vi "Generate Simulated Data.vi"(6 "Acquisition":refnum<queue>, 8 "error in (no error)":errorcluster, 11 "Data Stream":dbl[](array[numeric])) -> (0 "error out":errorcluster, 2 "Data Out":variant[](array[variant]), 3 "Disconnected":bool=TRUE)   [LabVIEW 2022 SP3, in "Acquisition.lvlib"]
doc: "Generates sample waveforms according to the signal type in the HW Config input."
uses:
  Acquisition.lvlib
  support/Message Queue/Message Cluster.ctl
  <vilib>/Analysis/2dsp.llb/2D Convolution (DBL).vi
  support/Message Queue/Enqueue Message (Single).vi
  GlobalVariable/GlobalPowerByTime.vi
  GlobalVariable/GlobalSet0.vi
  GlobalVariable/GlobalPosYbyTime.vi
  GlobalVariable/GlobalPosXbyTime.vi
  GlobalVariable/GlobalProfileByTime.vi
  GlobalVariable/Globalt0.vi
  GlobalVariable/GlobalTensionByTime.vi
  GlobalVariable/GlobalTemperatureByTime.vi
  GlobalVariable/GlobalTimeStep.vi
  <vilib>/gmath/interp.llb/Create Mesh Grid (2D) (x,y arrays).vi
  support/Message Queue/Message Queue.lvlib
  <vilib>/gmath/NI_Gmath.lvlib
  <vilib>/Analysis/NI_AALPro.lvlib
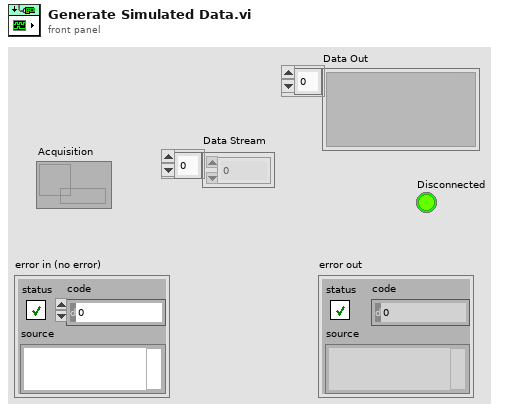
[diagram p1: front panel]
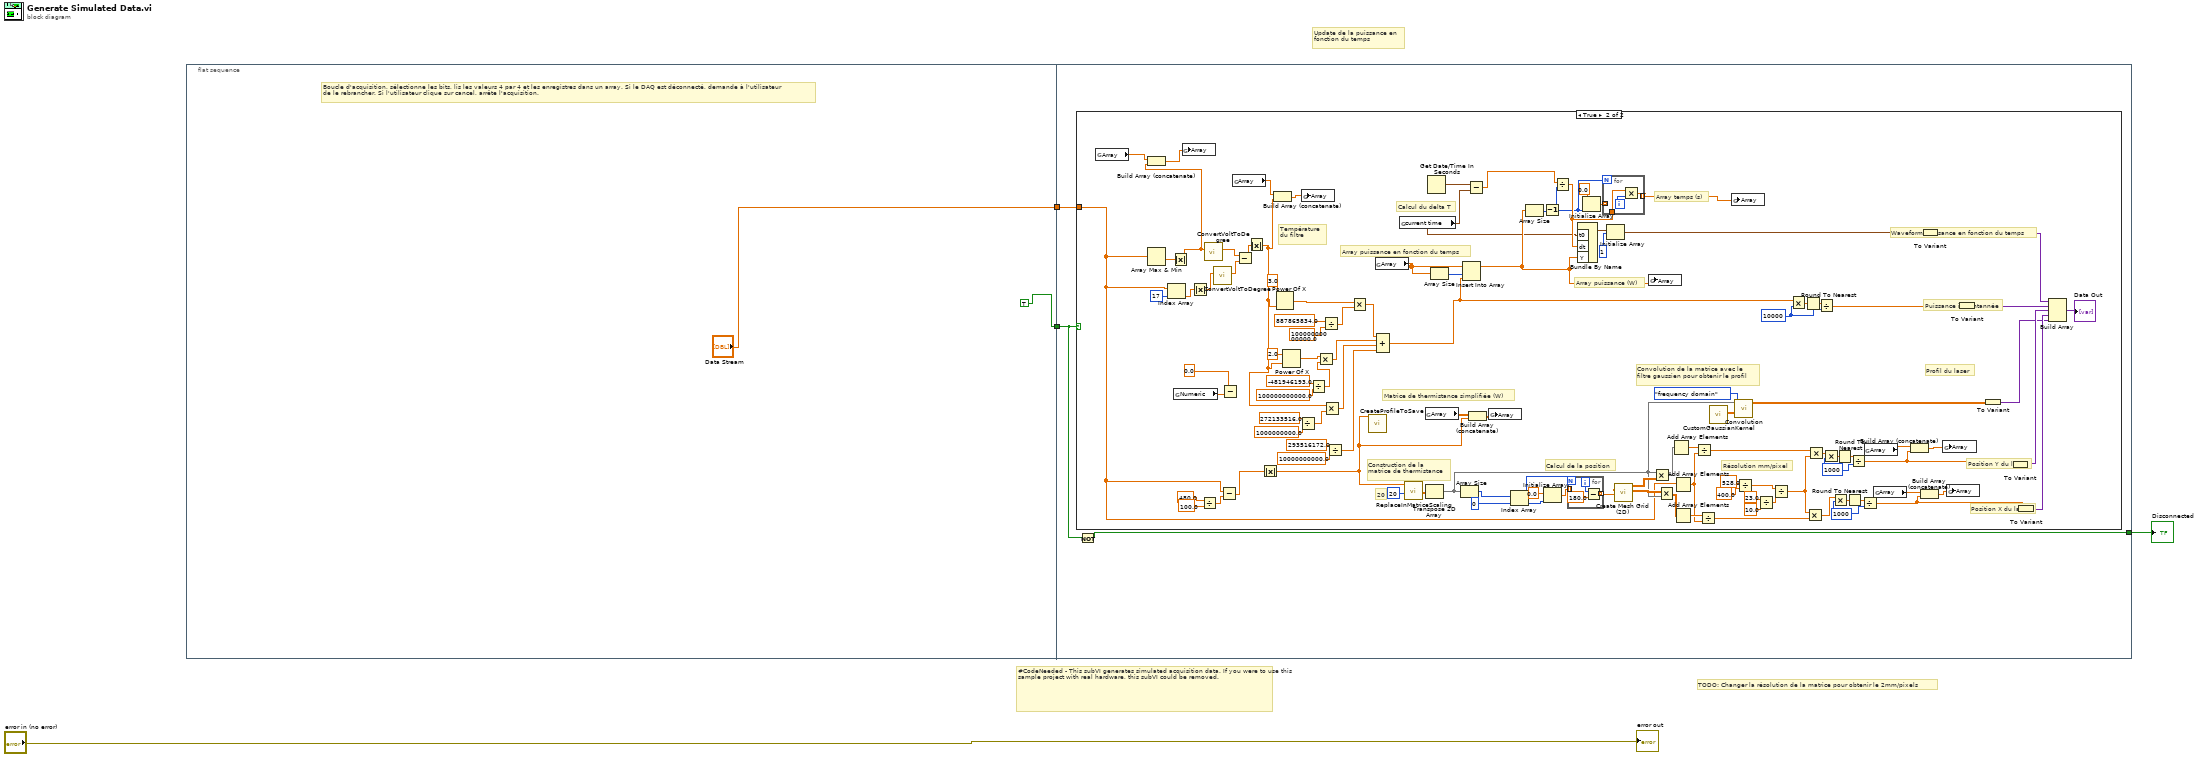
[diagram p0: block diagram]
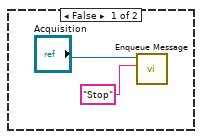
[diagram p2: hidden frame]
diagram:
  # "TODO: Changer la résolution de la matrice pour obtenir le 2mm/pixels"
  # "Update de la puissance en\nfonction du temps"
  # "#CodeNeeded - This subVI generates simulated acquisition data. If you were to use this sample project with real hardware, this subVI could be removed."
  n1 = flat-sequence {
    tunnel: [TRUE] -> w3
    tunnel: ["Data Stream"] -> w1
    tunnel: w3 -> [w7]
    tunnel: [w9] -> w2
    tunnel: w1 -> [w8]
    frame #0 {
      # "Boucle d'acquisition, sélectionne les bits, lis les valeurs 4 par 4 et les enregistres dans un array. Si le DAQ est déconnecté, demande à l'utilisateur \nde le rebrancher. Si l'utilisateur clique sur cancel, arrête l'acquisition."
    }
    frame #1 {
      n2 = case shown="True" w7 {
        tunnel: w8 -> [_ w42]
        frame False {
          n3 = call-poly "Enqueue Message.vi"("Message"="Stop", "Message Queue"="Acquisition") -> ()  [unwired: 8 in, 2 out]
        }
        frame True {
          w79 = 1000
          w83 = 1000
          w89 = 10000
          # "20"
          # "Résolution mm/pixel"
          # "Calcul du delta T"
          # "Matrice de thermistance simplifiée (W)"
          # "Température \ndu filtre"
          # "Calcul de la position"
          # "Construction de la \nmatrice de thermistance"
          # "Position X du laser"
          # "Position Y du laser"
          # "Profil du laser"
          # "Puissance instantannée"
          # "Waveform puissance en fonction du temps"
          # "Array puissance (W)"
          # "Array temps (s)"
          # "Convolution de la matrice avec le \nfiltre gaussien pour obtenir le profil"
          # "Array puissance en fonction du temps"
          n4 = global read "GlobalTensionByTime.vi" "Array"() -> (w59:dbl[])
          n5 = Array Max & Min(array=w42) -> (min value=w18:dbl)  [unwired: 3 out]
          n6 = Index Array(array=w42, index=17) -> (element=w17:dbl)
          n7 = Absolute Value(x=w18) -> (abs(x)=w41:dbl)
          n8 = Build Array (concatenate)(w59, w41) -> (w58:dbl[])
          n9 = global read "GlobalSet0.vi" "Numeric"() -> (w20:dbl)
          n10 = global write "GlobalTensionByTime.vi" "Array"(w58) -> ()
          n11 = Absolute Value(x=w17) -> (abs(x)=w16:dbl)
          n12 = Divide(x=480.0, y=100.0) -> (x/y=w48:dbl)
          n13 = call "ConvertVoltToDegree.vi"("Tension"=w41) -> ("Température"=w14:dbl)  [unwired: 10 in]
          n14 = call "ConvertVoltToDegree.vi"("Tension"=w16) -> ("Température"=w15:dbl)  [unwired: 10 in]
          n15 = Subtract(x=w42, y=w48) -> (x-y=w47:dbl[])
          n16 = Subtract(x=0.0, y=w20) -> ()  [unwired: 1 out]
          n17 = global read "GlobalTemperatureByTime.vi" "Array"() -> (w56:dbl[])
          n18 = Subtract(x=w14, y=w15) -> (x-y=w13:dbl)
          n19 = Absolute Value(x=w13) -> (abs(x)=w12:dbl)
          n20 = Absolute Value(x=w47) -> (abs(x)=w46:dbl[])
          n21 = Build Array (concatenate)(w56, w12) -> (w57:dbl[])
          n22 = Power Of X(1:w12, 2:3.0 ("y")) -> (0:w38:dbl)
          n23 = Power Of X(1:w12, 2:2.0 ("y")) -> (0:w32:dbl)
          n24 = Divide(x=272133516.0, y=1000000000.0) -> (x/y=w27:dbl)
          n25 = global write "GlobalTemperatureByTime.vi" "Array"(w57) -> ()
          n26 = Divide(x=-481946193.0, y=100000000000.0) -> (x/y=w31:dbl)
          n27 = Multiply(x=w32, y=w31) -> (x*y=w29:dbl)
          n28 = Divide(x=887865834.0, y=10000000000000.0) -> (x/y=w37:dbl)
          n29 = Multiply(x=w12, y=w27) -> (x*y=w26:dbl)
          n30 = Divide(x=293516172.0, y=10000000000.0) -> (x/y=w22:dbl)
          n31 = Multiply(x=w38, y=w37) -> (x*y=w34:dbl)
          n32 = call "CreateProfileToSave.vi"("Input Array"=w46) -> ()  [unwired: 10 in, 1 out]
          n33 = global read "GlobalPowerByTime.vi" "Array"() -> (w121:dbl[])
          n34 = Compound Arithmetic op=ADD(w34, w29, w26, w22) -> (w21:dbl)
          n35 = global read "Globalt0.vi" "current time"() -> (w61:timestamp)
          n36 = call "ReplaceInMatriceScaling.vi"("Input Scaling"=20, "Input Array"=w46) -> ("Output Array"=w116:dbl[][])  [unwired: 9 in]
          n37 = global read "GlobalProfileByTime.vi" "Array"() -> (w65:dbl[][])
          n38 = Transpose 2D Array(2D array=w116) -> (transposed array=w45:dbl[][])
          n39 = Get Date/Time In Seconds() -> (seconds since 1Jan1904=w62:timestamp)
          n40 = Array Size(array=w121) -> (size(s)=w120:i32)
          n41 = Array Size(array=w45) -> (size(s)=w110:i32[])
          n42 = Insert Into Array(array=w121, index=w120, new element=w21) -> (w74:dbl[])
          n43 = Subtract(x=w62, y=w61) -> (x-y=w60:dbl)
          n44 = Build Array (concatenate)(w65, w46) -> (w66:dbl[][])
          n45 = global write "GlobalProfileByTime.vi" "Array"(w66) -> ()
          n46 = Index Array(array=w110, index=0) -> (element=w105:i32)
          n47 = Array Size(array=w74) -> (size(s)=w64:i32)
          n48 = Decrement(x=w64) -> (x-1=w63:i32)
          n49 = Initialize Array(0.0 ("element"), w105) -> (w107:dbl[])
          n50 = Divide(x=w60, y=w63) -> (x/y=w114:dbl)
          n51 = for {
            N: w105 -> [_]
            tunnel: w107 -> [_] mode=indexing
            tunnel: [w122] -> w102 mode=indexing
            i -> [w123]
            n52 = Subtract(x=w123, y=180.0) -> (x-y=w122:dbl)
          }
          n53 = Bundle By Name("t0"=w61, "dt"=w114, "Y"=w74) -> (w118:waveform(dbl))  [unwired: 1 in]
          n54 = Initialize Array(0.0 ("element"), w63) -> (w112:dbl[])
          n55 = for {
            N: w63 -> [_]
            tunnel: w114 -> [w126]
            tunnel: w112 -> [_] mode=indexing
            tunnel: [w125] -> w73 mode=indexing
            i -> [w127]
            n56 = Multiply(x=w126, y=w127) -> (x*y=w125:dbl)
          }
          n57 = Initialize Array(w118, 1) -> (w93:waveform(dbl)[])
          n58 = call-poly <vilib>:"Create Mesh Grid (2D).vi"("y domain"=w102, "x domain"=w102) -> ("Y"=w101:dbl[][], "X"=w106:dbl[][])  [unwired: 7 in, 1 out]
          n59 = global write "GlobalPowerByTime.vi" "Array"(w74) -> ()
          n60 = Multiply(x=w45, y=w106) -> (x*y=w104:dbl[][])
          n61 = Multiply(x=w101, y=w45) -> (x*y=w100:dbl[][])
          n62 = Add Array Elements(numeric array=w104) -> (sum=w103:dbl)
          n63 = Add Array Elements(numeric array=w42) -> (sum=w98:dbl)
          n64 = Add Array Elements(numeric array=w100) -> (sum=w99:dbl)
          n65 = Divide(x=w103, y=w98) -> (x/y=w96:dbl)
          n66 = Divide(x=w99, y=w98) -> (x/y=w97:dbl)
          n67 = call "CustomGaussianKernel.vi"() -> ("array"=w111:dbl[][])  [unwired: 11 in]
          n68 = global write "GlobalTimeStep.vi" "Array"(w73) -> ()
          n69 = call-poly <vilib>:"Convolution.vi"("algorithm"=enum32{"direct", "frequency domain"}."frequency domain", "Y"=w111, "X"=w45) -> ("X * Y"=w44:dbl[][])  [unwired: 7 in, 1 out]
          n70 = Divide(x=528.0, y=400.0) -> (x/y=w53:dbl)
          n71 = Divide(x=23.0 ("y"), y=10.0) -> (x/y=w52:dbl)
          n72 = Divide(x=w53, y=w52) -> (x/y=w51:dbl)
          n73 = Multiply(x=w21, y=w89) -> (x*y=w90:dbl)
          n74 = Round To Nearest(number=w90) -> (nearest integer value=w88:dbl)
          n75 = Multiply(x=w51, y=w97) -> (x*y=w76:dbl)
          n76 = Multiply(x=w96, y=w51) -> (x*y=w80:dbl)
          n77 = Divide(x=w88, y=w89) -> (x/y=w84:dbl)
          n78 = Multiply(x=w80, y=w83) -> (x*y=w82:dbl)
          n79 = Multiply(x=w76, y=w79) -> (x*y=w78:dbl)
          n80 = Round To Nearest(number=w82) -> (nearest integer value=w81:dbl)
          n81 = Round To Nearest(number=w78) -> (nearest integer value=w77:dbl)
          n82 = Divide(x=w81, y=w83) -> (x/y=w67:dbl)
          n83 = Divide(x=w77, y=w79) -> (x/y=w71:dbl)
          n84 = global read "GlobalPosXbyTime.vi" "Array"() -> (w68:dbl[])
          n85 = global read "GlobalPosYbyTime.vi" "Array"() -> (w72:dbl[])
          n86 = Build Array (concatenate)(w68, w67) -> (w69:dbl[])
          n87 = Build Array (concatenate)(w72, w71) -> (w70:dbl[])
          n88 = To Variant(anything=w93) -> (Variant=w92:variant)
          n89 = global write "GlobalPosXbyTime.vi" "Array"(w69) -> ()
          n90 = global write "GlobalPosYbyTime.vi" "Array"(w70) -> ()
          n91 = To Variant(anything=w84) -> (Variant=w85:variant)
          n92 = To Variant(anything=w44) -> (Variant=w75:variant)
          n93 = To Variant(anything=w67) -> (Variant=w86:variant)
          n94 = To Variant(anything=w71) -> (Variant=w87:variant)
          n95 = Build Array(w92, w85, w86, w87, w75) -> (→"Data Out":variant[])
        }
      }
      n96 = Not(x=w7) -> (.not. x?=w9:bool)
    }
  }
  "error out" <- "error in (no error)"
  "Disconnected" <- w2
